vi "LoadConfig.vi"() -> (3 "Config":T1={"Pico"="COM5", "Range"=enum."0.26", "Mode"=enum."Serial", "R"=[0.19948381185531616, 0.39327406883239746, 0.3932740092277527]})   [LabVIEW 2025]
uses:
  Config.ctl
  Range.ctl
  Mode.ctl
  Globals.vi
panel:
  # "R1 Only"
  # "Serial"
  # "Parallel"
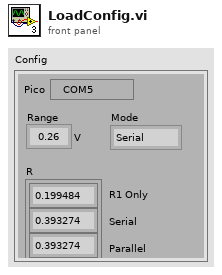
[diagram p1: front panel]
types:
  T1 = typedef "Config.ctl" = cluster{"Pico":refnum<visa-resource-name>, "Range":T2, "Mode":T3, "R":dbl[]}
  T2 = typedef "Range.ctl" = enum16{"0.26", "0.52", "1.03", "2.05", "4.1", "6.2"}
  T3 = typedef "Mode.ctl" = enum16{"R1 Only", "Parallel", "Serial"}
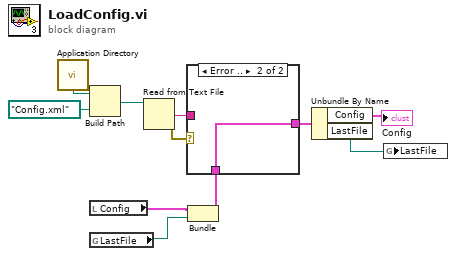
[diagram p0: block diagram]
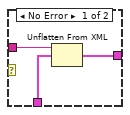
[diagram p2: hidden frame]
diagram:
  n1 = call <vilib>:"Application Directory.vi"() -> ("Application Directory"=w10:path)
  n2 = Build Path(base path=w10, name or relative path=path "Config.xml") -> (appended path=w9:path)
  n3 = local read "Config"() -> (w7:T1)
  n4 = global read "Globals.vi" "LastFile"() -> (w3:path)
  n5 = Read from Text File(file (use dialog)=w9) -> (text=w8:string, error out=w1:errorcluster)  [unwired: 3 in, 2 out]
  n6 = Bundle("Config"=w7, "LastFile"=w3) -> (w6:cluster{"Config":T1, "LastFile":path})  [unwired: 1 in]
  n7 = case shown="Error .." w1 {
    tunnel: w8 -> [w14 _]
    tunnel: w6 -> [w13 w15]
    tunnel: [w12 w15] -> w5
    frame No Error {
      n8 = Unflatten From XML(xml string=w14, type=w13) -> (value=w12:cluster{"Config":T1, "LastFile":path})  [unwired: 1 in, 1 out]
    }
    frame Error {
    }
  }
  n9 = Unbundle By Name(w5) -> ("Config"=→"Config":T1, "LastFile"=w2:path)
  n10 = global write "Globals.vi" "LastFile"(w2) -> ()
